vi "SVI_AL_Parser.vi"(4 "Cluster in":cluster{"Array":dbl[], "Array":dbl[]}, 6 "Time Step (ms)":i32, 7 "read buffer":string) -> (0 "Cluster out":cluster{"Array":dbl[], "Array":dbl[]}, 3 "Temperature (°C)":dbl)   [LabVIEW 2014]
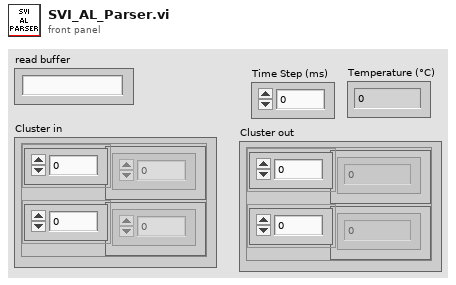
[diagram p1: front panel]
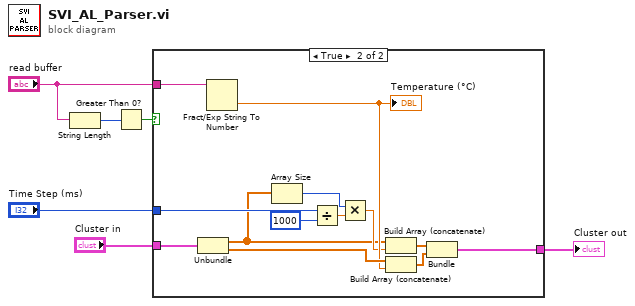
[diagram p0: block diagram]
diagram:
  n1 = String Length(string="read buffer") -> (length=w6:i32)
  n2 = Greater Than 0?(x=w6) -> (x > 0?=w5:bool)
  n3 = case shown="True" w5 {
    tunnel: "read buffer" -> [_ w15]
    tunnel: [w7 w19] -> w1
    tunnel: "Cluster in" -> [w7 w20]
    tunnel: "Time Step (ms)" -> [_ w10]
    frame False {
    }
    frame True {
      n4 = Unbundle(w20) -> ("Array"=w8:dbl[], "Array"=w16:dbl[])
      n5 = Fract/Exp String To Number(string=w15) -> (number=w13:dbl)  [unwired: 3 in, 1 out]
      "Temperature (°C)" <- w13
      n6 = Array Size(array=w8) -> (size(s)=w9:i32)
      n7 = Divide(x=w10, y=1000) -> (x/y=w12:dbl)
      n8 = Multiply(x=w9, y=w12) -> (x*y=w11:dbl)
      n9 = Build Array (concatenate)(w8, w11) -> (w18:dbl[])
      n10 = Build Array (concatenate)(w16, w13) -> (w17:dbl[])
      n11 = Bundle(w18, w17) -> (w19:cluster{dbl[], dbl[]})  [unwired: 1 in]
    }
  }
  "Cluster out" <- w1
